vi "Metrolab Digital Integrator Display.vi"(11 "Field":dbl[unit] format="%.4f") -> ()   [LabVIEW 2019]
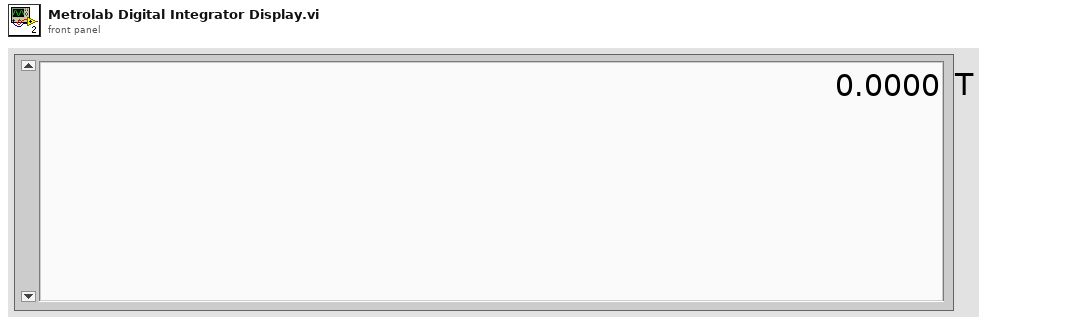
[diagram p1: front panel]
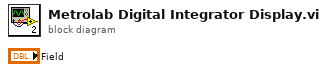
[diagram p0: block diagram]
diagram:
